vi "Write Hierarchy.vi"(8 "error in (no error)":errorcluster, 10 "Hierarchy":string[](array[string]), 11 "MetaDriver_v1 in":refnum<class "MetaDriver_v1.lvclass">) -> (0 "error out":errorcluster, 3 "MetaDriver_v1 out":refnum<class "MetaDriver_v1.lvclass">)   [LabVIEW 2020, in "MetaDriver_v1.lvclass"]
uses:
  MetaDriver_v1.lvclass
  MetaDriver_v1.lvclass/MetaDriver_v1.ctl
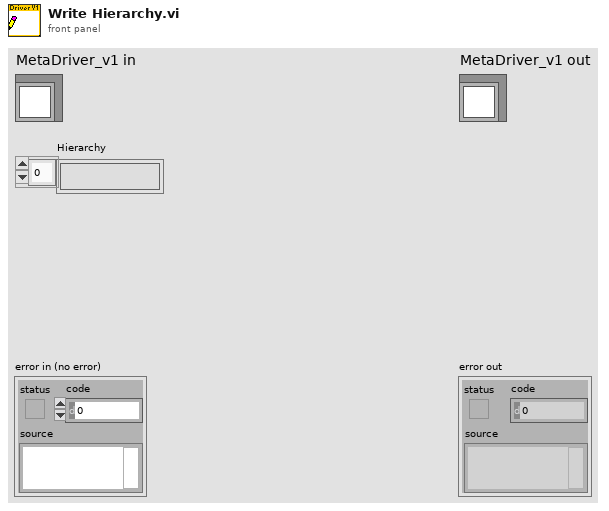
[diagram p1: front panel]
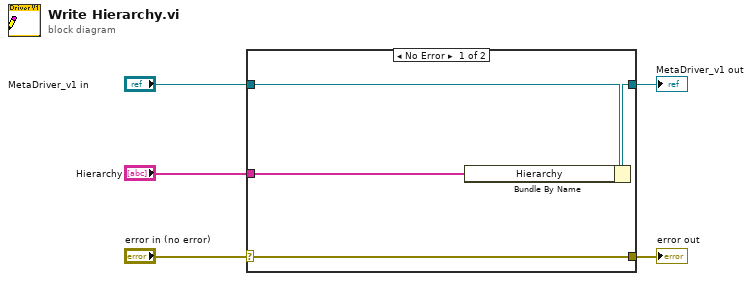
[diagram p0: block diagram]
diagram:
  n1 = case shown="No Error" "error in (no error)" {
    selector: "error in (no error)" -> [w9 w10]
    tunnel: [w9 w10] -> w4
    tunnel: [w7 w11] -> w2
    tunnel: "MetaDriver_v1 in" -> [w8 w11]
    tunnel: "Hierarchy" -> [w6 _]
    frame No Error {
      n2 = Bundle By Name(cluster=w8, "Hierarchy"=w6) -> (w7:refnum<class "MetaDriver_v1.lvclass">)
    }
    frame Error {
    }
  }
  "error out" <- w4
  "MetaDriver_v1 out" <- w2
